vi "PassFailWrite.vi"(7 "FailString":string, 8 "error in":errorcluster, 9 "End":string, 10 "PassString":string, 11 "TerminalIn":T1) -> (0 "error out":errorcluster, 3 "TerminalOut":T1)   [LabVIEW 2021, in "LibDan.lvlib"]
uses:
  LibDan.lvlib
  TerminalDef.ctl
  <vilib>/Utility/config.llb/Config Data RefNum.ctl
  <vilib>/Utility/config.llb/NI_LVConfig.lvlib
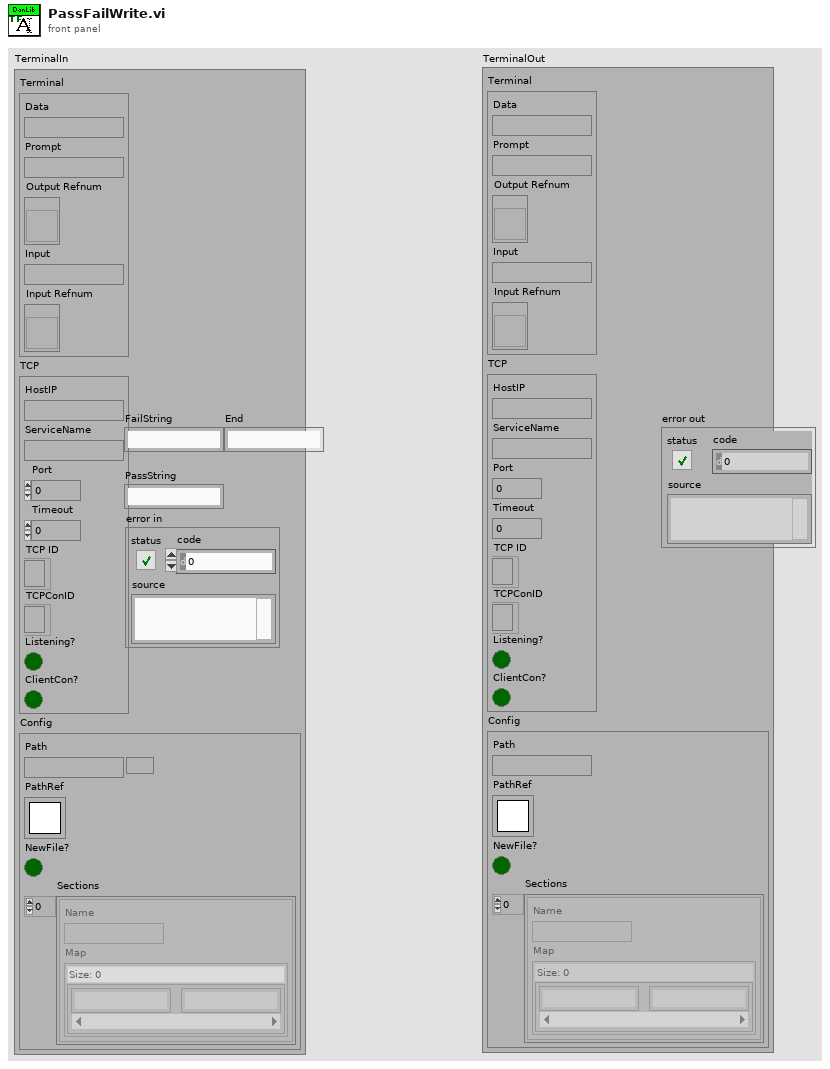
[diagram p1: front panel]
types:
  T1 = typedef "LibDan.lvlib/TerminalDef.ctl" = cluster{"Terminal":cluster{"Data":string, "Prompt":string, "Output Refnum":refnum<vi>, "Input":string, "Input Refnum":refnum<vi>}, "TCP":cluster{"HostIP":string, "ServiceName":string, "Port":u16, "Timeout":i32, "TCP ID":refnum<k5>, "TCPConID":refnum<k5>, "Listening?":bool, "ClientCon?":bool}, "Config":cluster{"Path":path, "PathRef":T2, "NewFile?":bool, "Sections":cluster{"Name":string, "Map":map{string, string}}[]}}
  T2 = typedef "NI_LVConfig.lvlib/Config Data RefNum.ctl" = refnum<k1>
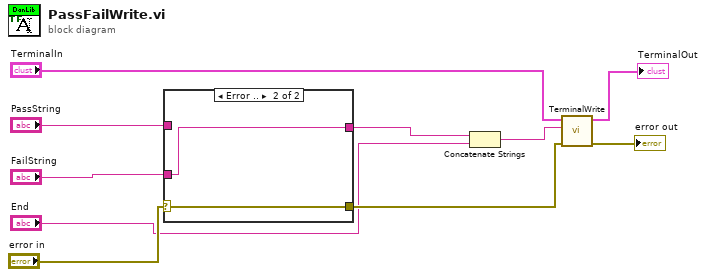
[diagram p0: block diagram]
diagram:
  n1 = case shown="Error .." "error in" {
    selector: "error in" -> [w12 w14]
    tunnel: [w12 w14] -> w6
    tunnel: "PassString" -> [w11 _]
    tunnel: "FailString" -> [_ w13]
    tunnel: [w11 w13] -> w2
    frame No Error {
    }
    frame Error {
    }
  }
  n2 = Concatenate Strings(w2, "End") -> (w3:string)
  n3 = call "TerminalWrite.vi"("error in"=w6, "string"=w3, "TerminalIn"="TerminalIn") -> ("error out"=→"error out":errorcluster, "TerminalOut"=→"TerminalOut":T1)  [unwired: 7 in]
